vi "CRYGet LevelUnit for Disp.vi"(10 "In Value":u16) -> (1 "Lvl Unit":i16)   [LabVIEW 2013]
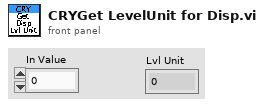
[diagram p1: front panel]
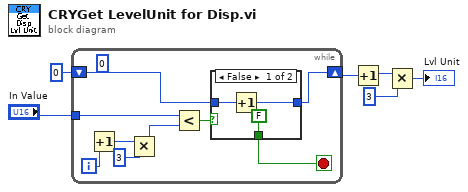
[diagram p0: block diagram]
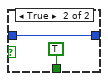
[diagram p2: hidden frame]
diagram:
  (unwired) u8 0
  n1 = while {
    shift-right: [w15] -> w4
    shift-left: i16 0 -> [w14]
    tunnel: "In Value" -> [w12]
    i -> [w11]
    stop <- w13 stop-if-true
    n2 = Increment(x=w11) -> (x+1=w9:i32)
    n3 = Multiply(x=w9, y=3) -> (x*y=w7:i32)
    n4 = Less?(x=w12, y=w7) -> (x < y?=w10:bool)
    n5 = case shown="False" w10 {
      tunnel: w14 -> [w18 w19]
      tunnel: [w16 w19] -> w15
      tunnel: [FALSE TRUE] -> w13
      frame False {
        n6 = Increment(x=w18) -> (x+1=w16:i16)
      }
      frame True {
      }
    }
  }
  n7 = Increment(x=w4) -> (x+1=w3:i16)
  n8 = Multiply(x=w3, y=i16 3) -> (x*y=→"Lvl Unit":i16)
